vi "Robo Team Send Error event.vi"(8 "error in (no error)":errorcluster) -> ()   [LabVIEW 2015]
uses:
  Robo Team Globals.vi
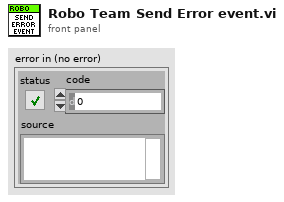
[diagram p1: front panel]
types:
  T1 = typedef "Robo System State Refs.ctl" = cluster{"Engage Motor":refnum<vi>, "Auto Level":refnum<vi>, "IMU led":refnum<vi>, "Evaluate Enable":refnum<vi>, "Motor Led":refnum<vi>, "Error Descript":refnum<vi>, "Error Led":refnum<vi>, "Error":refnum<vi>}
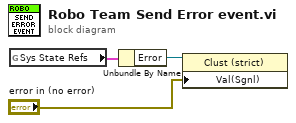
[diagram p0: block diagram]
diagram:
  n1 = global read "Robo Team Globals.vi" "Sys State Refs"() -> (w2:T1)
  n2 = Unbundle By Name(w2) -> ("Error"=w1:refnum<vi>)
  n3 = property class="Clust (strict)"(reference=w1, "Val(Sgnl)"="error in (no error)") -> ()  [unwired: 1 in, 2 out]
